vi "Send Set OD Entry Values.vi"(7 "Message Priority (Normal)":T2=enum."Normal", 8 "error in (no error)":errorcluster, 10 "Values":T1(array[cluster]) {"Multiplexer"."Index" format="%x"}, 11 "Message Enqueuer":refnum<class "Message Enqueuer.lvclass">) -> (0 "error out":errorcluster, 3 "Message Enqueuer out":refnum<class "Message Enqueuer.lvclass">)   [LabVIEW 2020, in "Object Dictionary UI.lvlib" / "Set OD Entry Values Msg.lvclass"]
doc: "This VI sends the message to an actor."
uses:
  Set OD Entry Values Msg.lvclass
  Set OD Entry Values Msg.lvclass/Set OD Entry Values Msg.ctl
  <vilib>/ActorFramework/Message Enqueuer/Message Enqueuer.lvclass
  <vilib>/ActorFramework/Message Enqueuer/Message Priority.ctl
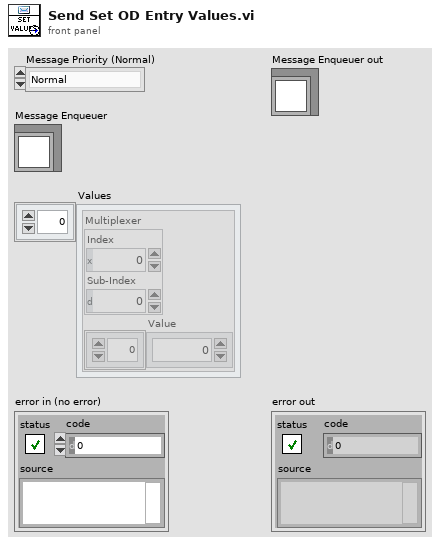
[diagram p1: front panel]
types:
  T1 = cluster{"Multiplexer":cluster{"Index":u16, "Sub-Index":i16}, "Value":u8[]}[]
  T2 = typedef "Actor Framework.lvlib/Message Enqueuer.lvclass/Message Priority.ctl" = enum16{"Low", "Normal", "High"}
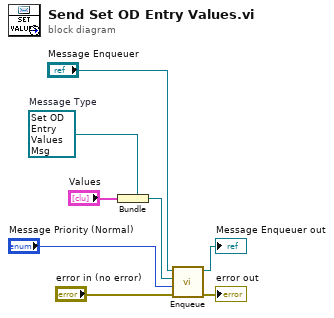
[diagram p0: block diagram]
diagram:
  w2 = refnum<class "Set OD Entry Values Msg.lvclass"> refnum  # Message Type
  n1 = Bundle(cluster=w2, "Values") -> (w3:refnum<class "Set OD Entry Values Msg.lvclass">)
  n2 = call <vilib>:"Enqueue.vi"("error in (no error)"="error in (no error)", "Message Priority (Normal)"="Message Priority (Normal)", "Message"=w3, "Message Enqueuer in"="Message Enqueuer") -> ("error out"=→"error out":errorcluster, "Message Enqueuer out"=→"Message Enqueuer out":refnum<class "Message Enqueuer.lvclass">)  [unwired: 6 in]
